vi "UTILITY Integral.vi"(8 "Error In":errorcluster, 10 "dt":dbl=1.0, 11 "Array Input":dbl[](array[numeric])) -> (0 "Error Out":errorcluster, 3 "Integral":dbl)   [LabVIEW 2023]
uses:
  <vilib>/Analysis/2dsp.llb/Integral Method.ctl
  <vilib>/Analysis/NI_AALPro.lvlib
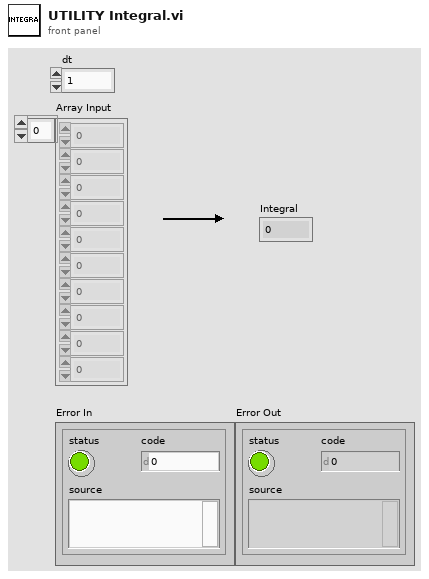
[diagram p1: front panel]
types:
  T1 = typedef "NI_AALPro.lvlib/Integral Method.ctl" = i32
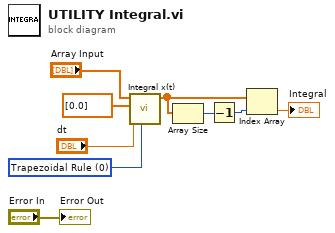
[diagram p0: block diagram]
diagram:
  w7 = T1 0 items=["Trapezoidal Rule", "Simpson's Rule", "Simpson's 3/8 Rule", "Bode Rule"] ("integration method")
  n1 = call <vilib>:"Integral x(t).vi"("integration method"=w7, "dt"="dt", "Initial Condition"=dbl[] [0.0], "X"="Array Input") -> ("Integral X"=w6:dbl[])  [unwired: 6 in, 1 out]
  n2 = Array Size(array=w6) -> (size(s)=w4:i32)
  n3 = Decrement(x=w4) -> (x-1=w3:i32)
  n4 = Index Array(array=w6, index=w3) -> (element=→"Integral":dbl)
  "Error Out" <- "Error In"
